vi "GeoData.vi"() -> ()   [LabVIEW 2017] (continued)
Washington Parish\tH1\n71075\t22119\tSpringhill\tLA\tWebster Parish\tH1\n71067\t22119\tPrinceton\tLA\tWebster Parish\tH1\n71071\t22119\tSarepta\tLA\tWebster Parish\tH1\n71038\t22119\tHaynesville\tLA\tWebster Parish\tH1\n71073\t22119\tSibley\tLA\tWebster Parish\tH1\n71024\t22119\tDubberly\tLA\tWebster Parish\tH1\n71055\t22119\tMinden\tLA\tWebster Parish\tH1\n71072\t22119\tShongaloo\tLA\tWebster Parish\tH1\n71039\t22119\tHeflin\tLA\tWebster Parish\tH1\n71037\t22119\tHaughton\tLA\tWebster Parish\tH1\n71023\t22119\tDoyline\tLA\tWebster Parish\tH1\n71021\t22119\tCullen\tLA\tWebster Parish\tH1\n71018\t22119\tCotton valley\tLA\tWebster Parish\tH1\n70773\t22121\tRougon\tLA\tWest Baton Rouge Parish\tH1\n70710\t22121\tAddis\tLA\tWest Baton Rouge Parish\tH1\n70764\t22121\tPlaquemine\tLA\tWest Baton Rouge Parish\tH1\n70736\t22121\tGlynn\tLA\tWest Baton Rouge Parish\tH1\n70719\t22121\tBrusly\tLA\tWest Baton Rouge Parish\tH1\n70767\t22121\tPort allen\tLA\tWest Baton Rouge Parish\tH1\n70729\t22121\tErwinville\tLA\tWest Baton Rouge Parish\tH1\n71263\t22123\tOak grove\tLA\tWest Carroll Parish\tH1\n71269\t22123\tRayville\tLA\tWest Carroll Parish\tH1\n71286\t22123\tTransylvania\tLA\tWest Carroll Parish\tH1\n71253\t22123\tKilbourne\tLA\tWest Carroll Parish\tH1\n71266\t22123\tPioneer\tLA\tWest Carroll Parish\tH1\n71237\t22123\tEpps\tLA\tWest Carroll Parish\tH1\n71242\t22123\tForest\tLA\tWest Carroll Parish\tH1\n70748\t22125\tJackson\tLA\tWest Feliciana Parish\tH1\n70787\t22125\tWeyanoke\tLA\tWest Feliciana Parish\tH1\n70775\t22125\tSaint francisville\tLA\tWest Feliciana Parish\tH1\n70712\t22125\tAngola\tLA\tWest Feliciana Parish\tH1\n70784\t22125\tWakefield\tLA\tWest Feliciana Parish\tH1\n70782\t22125\tTunica\tLA\tWest Feliciana Parish\tH1\n71070\t22127\tSaline\tLA\tWinn Parish\tH1\n71483\t22127\tWinnfield\tLA\tWinn Parish\tH1\n71479\t22127\tTullos\tLA\tWinn Parish\tH1\n71465\t22127\tOlla\tLA\tWinn Parish\tH1\n71471\t22127\tSaint maurice\tLA\tWinn Parish\tH1\n71457\t22127\tNatchitoches\tLA\tWinn Parish\tH1\n71031\t22127\tGoldonna\tLA\tWinn Parish\tH1\n71422\t22127\tDodson\tLA\tWinn Parish\tH1\n71404\t22127\tAtlanta\tLA\tWinn Parish\tH1\n71454\t22127\tMontgomery\tLA\tWinn Parish\tH1\n71432\t22127\tGeorgetown\tLA\tWinn Parish\tH1\n71473\t22127\tSikes\tLA\tWinn Parish\tH1\n71440\t22127\tJoyce\tLA\tWinn Parish\tH1\n71410\t22127\tCalvin\tLA\tWinn Parish\tH1\n4212\t23001\tAuburn\tME\tAndroscoggin County\tH1\n4220\t23001\tBuckfield\tME\tAndroscoggin County\tH1\n4240\t23001\tLewiston\tME\tAndroscoggin County\tH1\n4274\t23001\tPoland\tME\tAndroscoggin County\tH1\n4270\t23001\tOxford\tME\tAndroscoggin County\tH1\n4256\t23001\tMechanic falls\tME\tAndroscoggin County\tH1\n4239\t23001\tJay\tME\tAndroscoggin County\tH1\n4230\t23001\tEast poland\tME\tAndroscoggin County\tH1\n4228\t23001\tEast livermore\tME\tAndroscoggin County\tH1\n4210\t23001\tAuburn\tME\tAndroscoggin County\tH1\n4222\t23001\tDurham\tME\tAndroscoggin County\tH1\n4254\t23001\tLivermore falls\tME\tAndroscoggin County\tH1\n4252\t23001\tLisbon falls\tME\tAndroscoggin County\tH1\n4211\t23001\tAuburn\tME\tAndroscoggin County\tH1\n4238\t23001\tHebron\tME\tAndroscoggin County\tH1\n4266\t23001\tNorth turner\tME\tAndroscoggin County\tH1\n4288\t23001\tWest minot\tME\tAndroscoggin County\tH1\n4260\t23001\tNew gloucester\tME\tAndroscoggin County\tH1\n4250\t23001\tLisbon\tME\tAndroscoggin County\tH1\n4280\t23001\tSabattus\tME\tAndroscoggin County\tH1\n4263\t23001\tLeeds\tME\tAndroscoggin County\tH1\n4253\t23001\tLivermore\tME\tAndroscoggin County\tH1\n4243\t23001\tLewiston\tME\tAndroscoggin County\tH1\n4282\t23001\tTurner\tME\tAndroscoggin County\tH1\n4258\t23001\tMinot\tME\tAndroscoggin County\tH1\n4291\t23001\tWest poland\tME\tAndroscoggin County\tH1\n4223\t23001\tDanville\tME\tAndroscoggin County\tH1\n4236\t23001\tGreene\tME\tAndroscoggin County\tH1\n4241\t23001\tLewiston\tME\tAndroscoggin County\tH1\n4487\t23003\tSpringfield\tME\tAroostook County\tH1\n4739\t23003\tEagle lake\tME\tAroostook County\tH1\n4733\t23003\tBenedicta\tME\tAroostook County\tH1\n4775\t23003\tSheridan\tME\tAroostook County\tH1\n4762\t23003\tNew sweden\tME\tAroostook County\tH1\n4459\t23003\tMattawamkeag\tME\tAroostook County\tH1\n4777\t23003\tStacyville\tME\tAroostook County\tH1\n4761\t23003\tNew limerick\tME\tAroostook County\tH1\n4750\t23003\tLimestone\tME\tAroostook County\tH1\n4787\t23003\tWestfield\tME\tAroostook County\tH1\n4740\t23003\tEaston\tME\tAroostook County\tH1\n4746\t23003\tGrand isle\tME\tAroostook County\tH1\n4763\t23003\tOakfield\tME\tAroostook County\tH1\n4776\t23003\tSherman\tME\tAroostook County\tH1\n4738\t23003\tCrouseville\tME\tAroostook County\tH1\n4772\t23003\tSaint agatha\tME\tAroostook County\tH1\n4764\t23003\tOxbow\tME\tAroostook County\tH1\n4745\t23003\tFrenchville\tME\tAroostook County\tH1\n4424\t23003\tDanforth\tME\tAroostook County\tH1\n4742\t23003\tFort fairfield\tME\tAroostook County\tH1\n4736\t23003\tCaribou\tME\tAroostook County\tH1\n4756\t23003\tMadawaska\tME\tAroostook County\tH1\n4779\t23003\tSinclair\tME\tAroostook County\tH1\n4783\t23003\tStockholm\tME\tAroostook County\tH1\n4751\t23003\tLimestone\tME\tAroostook County\tH1\n4735\t23003\tBridgewater\tME\tAroostook County\tH1\n4732\t23003\tAshland\tME\tAroostook County\tH1\n4743\t23003\tFort kent\tME\tAroostook County\tH1\n4757\t23003\tMapleton\tME\tAroostook County\tH1\n4786\t23003\tWashburn\tME\tAroostook County\tH1\n4769\t23003\tPresque isle\tME\tAroostook County\tH1\n4781\t23003\tWallagrass\tME\tAroostook County\tH1\n4451\t23003\tKingman\tME\tAroostook County\tH1\n4747\t23003\tIsland falls\tME\tAroostook County\tH1\n4768\t23003\tPortage\tME\tAroostook County\tH1\n4744\t23003\tFort kent mills\tME\tAroostook County\tH1\n4737\t23003\tClayton lake\tME\tAroostook County\tH1\n4497\t23003\tWytopitlock\tME\tAroostook County\tH1\n4730\t23003\tHoulton\tME\tAroostook County\tH1\n4758\t23003\tMars hill\tME\tAroostook County\tH1\n4471\t23003\tOrient\tME\tAroostook County\tH1\n4766\t23003\tPerham\tME\tAroostook County\tH1\n4773\t23003\tSaint david\tME\tAroostook County\tH1\n4760\t23003\tMonticello\tME\tAroostook County\tH1\n4785\t23003\tVan buren\tME\tAroostook County\tH1\n4780\t23003\tSmyrna mills\tME\tAroostook County\tH1\n4774\t23003\tSaint francis\tME\tAroostook County\tH1\n4734\t23003\tBlaine\tME\tAroostook County\tH1\n4062\t23005\tWindham\tME\tCumberland County\tH1\n4015\t23005\tCasco\tME\tCumberland County\tH1\n4093\t23005\tBuxton\tME\tCumberland County\tH1\n4109\t23005\tPortland\tME\tCumberland County\tH1\n4274\t23005\tPoland\tME\tCumberland County\tH1\n4078\t23005\tSouth freeport\tME\tCumberland County\tH1\n4082\t23005\tSouth windham\tME\tCumberland County\tH1\n4071\t23005\tRaymond\tME\tCumberland County\tH1\n4088\t23005\tWaterford\tME\tCumberland County\tH1\n4069\t23005\tPownal\tME\tCumberland County\tH1\n4098\t23005\tWestbrook\tME\tCumberland County\tH1\n4091\t23005\tWest baldwin\tME\tCumberland County\tH1\n4021\t23005\tCumberland center\tME\tCumberland County\tH1\n4222\t23005\tDurham\tME\tCumberland County\tH1\n4066\t23005\tOrrs island\tME\tCumberland County\tH1\n4034\t23005\tFreeport\tME\tCumberland County\tH1\n4033\t23005\tFreeport\tME\tCumberland County\tH1\n4040\t23005\tHarrison\tME\tCumberland County\tH1\n4096\t23005\tYarmouth\tME\tCumberland County\tH1\n4074\t23005\tScarborough\tME\tCumberland County\tH1\n4103\t23005\tPortland\tME\tCumberland County\tH1\n4105\t23005\tFalmouth\tME\tCumberland County\tH1\n4108\t23005\tPeaks island\tME\tCumberland County\tH1\n4110\t23005\tCumberland foreside\tME\tCumberland County\tH1\n4085\t23005\tSteep falls\tME\tCumberland County\tH1\n4123\t23005\tPortland\tME\tCumberland County\tH1\n4009\t23005\tBridgton\tME\tCumberland County\tH1\n4092\t23005\tWestbrook\tME\tCumberland County\tH1\n4079\t23005\tHarpswell\tME\tCumberland County\tH1\n4102\t23005\tPortland\tME\tCumberland County\tH1\n4097\t23005\tNorth yarmouth\tME\tCumberland County\tH1\n4038\t23005\tGorham\tME\tCumberland County\tH1\n4039\t23005\tGray\tME\tCumberland County\tH1\n4029\t23005\tSebago\tME\tCumberland County\tH1\n4101\t23005\tPortland\tME\tCumberland County\tH1\n4260\t23005\tNew gloucester\tME\tCumberland County\tH1\n4017\t23005\tChebeague island\tME\tCumberland County\tH1\n4070\t23005\tScarborough\tME\tCumberland County\tH1\n4116\t23005\tSouth portland\tME\tCumberland County\tH1\n4057\t23005\tNorth bridgton\tME\tCumberland County\tH1\n4077\t23005\tSouth casco\tME\tCumberland County\tH1\n4055\t23005\tNaples\tME\tCumberland County\tH1\n4106\t23005\tSouth portland\tME\tCumberland County\tH1\n4107\t23005\tCape elizabeth\tME\tCumberland County\tH1\n4122\t23005\tPortland\tME\tCumberland County\tH1\n4024\t23005\tEast baldwin\tME\tCumberland County\tH1\n4124\t23005\tPortland\tME\tCumberland County\tH1\n4013\t23005\tBustins island\tME\tCumberland County\tH1\n4019\t23005\tCliff island\tME\tCumberland County\tH1\n4050\t23005\tLong island\tME\tCumberland County\tH1\n4011\t23005\tBrunswick\tME\tCumberland County\tH1\n4032\t23005\tFreeport\tME\tCumberland County\tH1\n4064\t23005\tOld orchard beach\tME\tCumberland County\tH1\n4084\t23005\tStandish\tME\tCumberland County\tH1\n4112\t23005\tPortland\tME\tCumberland County\tH1\n4003\t23005\tBailey island\tME\tCumberland County\tH1\n4104\t23005\tPortland\tME\tCumberland County\tH1\n4984\t23007\tTemple\tME\tFranklin County\tH1\n4262\t23007\tNorth jay\tME\tFranklin County\tH1\n4225\t23007\tDryden\tME\tFranklin County\tH1\n4940\t23007\tFarmington falls\tME\tFranklin County\tH1\n4294\t23007\tWilton\tME\tFranklin County\tH1\n4239\t23007\tJay\tME\tFranklin County\tH1\n4966\t23007\tPhillips\tME\tFranklin County\tH1\n4938\t23007\tFarmington\tME\tFranklin County\tH1\n4285\t23007\tWeld\tME\tFranklin County\tH1\n4970\t23007\tRangeley\tME\tFranklin County\tH1\n4964\t23007\tOquossoc\tME\tFranklin County\tH1\n4961\t23007\tNew portland\tME\tFranklin County\tH1\n4983\t23007\tStrong\tME\tFranklin County\tH1\n4956\t23007\tNew vineyard\tME\tFranklin County\tH1\n4234\t23007\tEast wilton\tME\tFranklin County\tH1\n4224\t23007\tDixfield\tME\tFranklin County\tH1\n4227\t23007\tEast dixfield\tME\tFranklin County\tH1\n4982\t23007\tStratton\tME\tFranklin County\tH1\n4992\t23007\tWest farmington\tME\tFranklin County\tH1\n4955\t23007\tNew sharon\tME\tFranklin County\tH1\n4947\t23007\tKingfield\tME\tFranklin County\tH1\n4936\t23007\tEustis\tME\tFranklin County\tH1\n4616\t23009\tBrooklin\tME\tHancock County\tH1\n4660\t23009\tMount desert\tME\tHancock County\tH1\n4642\t23009\tHarborside\tME\tHancock County\tH1\n4646\t23009\tIslesford\tME\tHancock County\tH1\n4609\t23009\tBar harbor\tME\tHancock County\tH1\n4622\t23009\tCherryfield\tME\tHancock County\tH1\n4677\t23009\tSorrento\tME\tHancock County\tH1\n4408\t23009\tAurora\tME\tHancock County\tH1\n4679\t23009\tSouthwest harbor\tME\tHancock County\tH1\n4612\t23009\tBernard\tME\tHancock County\tH1\n4669\t23009\tProspect harbor\tME\tHancock County\tH1\n4629\t23009\tEast blue hill\tME\tHancock County\tH1\n4676\t23009\tSedgwick\tME\tHancock County\tH1\n4674\t23009\tSeal cove\tME\tHancock County\tH1\n4614\t23009\tBlue hill\tME\tHancock County\tH1\n4617\t23009\tBrooksville\tME\tHancock County\tH1\n4607\t23009\tGouldsboro\tME\tHancock County\tH1\n4673\t23009\tSargentville\tME\tHancock County\tH1\n4624\t23009\tCorea\tME\tHancock County\tH1\n4416\t23009\tBucksport\tME\tHancock County\tH1\n4476\t23009\tPenobscot\tME\tHancock County\tH1\n4684\t23009\tSurry\tME\tHancock County\tH1\n4675\t23009\tSeal harbor\tME\tHancock County\tH1\n4613\t23009\tBirch harbor\tME\tHancock County\tH1\n4650\t23009\tLittle deer isle\tME\tHancock County\tH1\n4431\t23009\tEast orland\tME\tHancock County\tH1\n4627\t23009\tDeer isle\tME\tHancock County\tH1\n4640\t23009\tHancock\tME\tHancock County\tH1\n4653\t23009\tBass harbor\tME\tHancock County\tH1\n4685\t23009\tSwans island\tME\tHancock County\tH1\n4644\t23009\tHulls cove\tME\tHancock County\tH1\n4672\t23009\tSalsbury cove\tME\tHancock County\tH1\n4605\t23009\tEllsworth\tME\tHancock County\tH1\n4681\t23009\tStonington\tME\tHancock County\tH1\n4421\t23009\tCastine\tME\tHancock County\tH1\n4664\t23009\tSullivan\tME\tHancock County\tH1\n4625\t23009\tCranberry isles\tME\tHancock County\tH1\n4429\t23009\tHolden\tME\tHancock County\tH1\n4472\t23009\tOrland\tME\tHancock County\tH1\n4634\t23009\tFranklin\tME\tHancock County\tH1\n4420\t23009\tCastine\tME\tHancock County\tH1\n4683\t23009\tSunset\tME\tHancock County\tH1\n4693\t23009\tWinter harbor\tME\tHancock County\tH1\n4662\t23009\tNortheast harbor\tME\tHancock County\tH1\n4635\t23009\tFrenchboro\tME\tHancock County\tH1\n4345\t23011\tGardiner\tME\tKennebec County\tH1\n4338\t23011\tAugusta\tME\tKennebec County\tH1\n4918\t23011\tBelgrade lakes\tME\tKennebec County\tH1\n4935\t23011\tEast vassalboro\tME\tKennebec County\tH1\n4353\t23011\tWhitefield\tME\tKennebec County\tH1\n4333\t23011\tAugusta\tME\tKennebec County\tH1\n4254\t23011\tLivermore falls\tME\tKennebec County\tH1\n4287\t23011\tBowdoin\tME\tKennebec County\tH1\n4364\t23011\tWinthrop\tME\tKennebec County\tH1\n4350\t23011\tLitchfield\tME\tKennebec County\tH1\n4346\t23011\tRandolph\tME\tKennebec County\tH1\n4910\t23011\tAlbion\tME\tKennebec County\tH1\n4989\t23011\tVassalboro\tME\tKennebec County\tH1\n4937\t23011\tFairfield\tME\tKennebec County\tH1\n4359\t23011\tSouth gardiner\tME\tKennebec County\tH1\n4284\t23011\tWayne\tME\tKennebec County\tH1\n4926\t23011\tChina village\tME\tKennebec County\tH1\n4351\t23011\tManchester\tME\tKennebec County\tH1\n4988\t23011\tUnity\tME\tKennebec County\tH1\n4927\t23011\tClinton\tME\tKennebec County\tH1\n4259\t23011\tMonmouth\tME\tKennebec County\tH1\n4363\t23011\tWindsor\tME\tKennebec County\tH1\n4355\t23011\tReadfield\tME\tKennebec County\tH1\n4360\t23011\tVienna\tME\tKennebec County\tH1\n4901\t23011\tWaterville\tME\tKennebec County\tH1\n4332\t23011\tAugusta\tME\tKennebec County\tH1\n4349\t23011\tKents hill\tME\tKennebec County\tH1\n4903\t23011\tWaterville\tME\tKennebec County\tH1\n4962\t23011\tNorth vassalboro\tME\tKennebec County\tH1\n4357\t23011\tRichmond\tME\tKennebec County\tH1\n4358\t23011\tSouth china\tME\tKennebec County\tH1\n4963\t23011\tOakland\tME\tKennebec County\tH1\n4978\t23011\tSmithfield\tME\tKennebec County\tH1\n4352\t23011\tMount vernon\tME\tKennebec County\tH1\n4265\t23011\tNorth monmouth\tME\tKennebec County\tH1\n4343\t23011\tEast winthrop\tME\tKennebec County\tH1\n4336\t23011\tAugusta\tME\tKennebec County\tH1\n4330\t23011\tAugusta\tME\tKennebec County\tH1\n4344\t23011\tFarmingdale\tME\tKennebec County\tH1\n4347\t23011\tHallowell\tME\tKennebec County\tH1\n4917\t23011\tBelgrade\tME\tKennebec County\tH1\n4856\t23013\tRockport\tME\tKnox County\tH1\n4949\t23013\tLiberty\tME\tKnox County\tH1\n4547\t23013\tFriendship\tME\tKnox County\tH1\n4847\t23013\tHope\tME\tKnox County\tH1\n4863\t23013\tVinalhaven\tME\tKnox County\tH1\n4865\t23013\tWest rockport\tME\tKnox County\tH1\n4860\t23013\tTenants harbor\tME\tKnox County\tH1\n4843\t23013\tCamden\tME\tKnox County\tH1\n4853\t23013\tNorth haven\tME\tKnox County\tH1\n4572\t23013\tWaldoboro\tME\tKnox County\tH1\n4563\t23013\tCushing\tME\tKnox County\tH1\n4862\t23013\tUnion\tME\tKnox County\tH1\n4574\t23013\tWashington\tME\tKnox County\tH1\n4645\t23013\tIsle au haut\tME\tKnox County\tH1\n4841\t23013\tRockland\tME\tKnox County\tH1\n4861\t23013\tThomaston\tME\tKnox County\tH1\n4855\t23013\tPort clyde\tME\tKnox County\tH1\n4858\t23013\tSouth thomaston\tME\tKnox County\tH1\n4851\t23013\tMatinicus\tME\tKnox County\tH1\n4854\t23013\tOwls head\tME\tKnox County\tH1\n4864\t23013\tWarren\tME\tKnox County\tH1\n4859\t23013\tSpruce head\tME\tKnox County\tH1\n4539\t23015\tBristol\tME\tLincoln County\tH1\n4543\t23015\tDamariscotta\tME\tLincoln County\tH1\n4348\t23015\tJefferson\tME\tLincoln County\tH1\n4353\t23015\tWhitefield\tME\tLincoln County\tH1\n4556\t23015\tEdgecomb\tME\tLincoln County\tH1\n4342\t23015\tDresden\tME\tLincoln County\tH1\n4554\t23015\tNew harbor\tME\tLincoln County\tH1\n4571\t23015\tTrevett\tME\tLincoln County\tH1\n4575\t23015\tWest boothbay harbor\tME\tLincoln County\tH1\n4852\t23015\tMonhegan\tME\tLincoln County\tH1\n4535\t23015\tAlna\tME\tLincoln County\tH1\n4570\t23015\tSquirrel island\tME\tLincoln County\tH1\n4537\t23015\tBoothbay\tME\tLincoln County\tH1\n4541\t23015\tChamberlain\tME\tLincoln County\tH1\n4544\t23015\tEast boothbay\tME\tLincoln County\tH1\n4573\t23015\tWalpole\tME\tLincoln County\tH1\n4354\t23015\tPalermo\tME\tLincoln County\tH1\n4572\t23015\tWaldoboro\tME\tLincoln County\tH1\n4862\t23015\tUnion\tME\tLincoln County\tH1\n4551\t23015\tBremen\tME\tLincoln County\tH1\n4558\t23015\tPemaquid\tME\tLincoln County\tH1\n4538\t23015\tBoothbay harbor\tME\tLincoln County\tH1\n4555\t23015\tNobleboro\tME\tLincoln County\tH1\n4568\t23015\tSouth bristol\tME\tLincoln County\tH1\n4576\t23015\tSouthport\tME\tLincoln County\tH1\n4564\t23015\tRound pond\tME\tLincoln County\tH1\n4341\t23015\tCoopers mills\tME\tLincoln County\tH1\n4553\t23015\tNewcastle\tME\tLincoln County\tH1\n4578\t23015\tWiscasset\tME\tLincoln County\tH1\n4864\t23015\tWarren\tME\tLincoln County\tH1\n4220\t23017\tBuckfield\tME\tOxford County\tH1\n4276\t23017\tRumford\tME\tOxford County\tH1\n4268\t23017\tNorway\tME\tOxford County\tH1\n4270\t23017\tOxford\tME\tOxford County\tH1\n4275\t23017\tRoxbury\tME\tOxford County\tH1\n4226\t23017\tEast andover\tME\tOxford County\tH1\n4267\t23017\tNorth waterford\tME\tOxford County\tH1\n4016\t23017\tCenter lovell\tME\tOxford County\tH1\n4051\t23017\tLovell\tME\tOxford County\tH1\n4088\t23017\tWaterford\tME\tOxford County\tH1\n4239\t23017\tJay\tME\tOxford County\tH1\n4221\t23017\tCanton\tME\tOxford County\tH1\n4261\t23017\tNewry\tME\tOxford County\tH1\n4041\t23017\tHiram\tME\tOxford County\tH1\n4289\t23017\tWest paris\tME\tOxford County\tH1\n4040\t23017\tHarrison\tME\tOxford County\tH1\n4224\t23017\tDixfield\tME\tOxford County\tH1\n4231\t23017\tStoneham\tME\tOxford County\tH1\n4292\t23017\tSumner\tME\tOxford County\tH1\n4238\t23017\tHebron\tME\tOxford County\tH1\n4009\t23017\tBridgton\tME\tOxford County\tH1\n4257\t23017\tMexico\tME\tOxford County\tH1\n4290\t23017\tPeru\tME\tOxford County\tH1\n4219\t23017\tBryant pond\tME\tOxford County\tH1\n4216\t23017\tAndover\tME\tOxford County\tH1\n4217\t23017\tBethel\tME\tOxford County\tH1\n4255\t23017\tGreenwood\tME\tOxford County\tH1\n4237\t23017\tHanover\tME\tOxford County\tH1\n4271\t23017\tParis\tME\tOxford County\tH1\n4037\t23017\tFryeburg\tME\tOxford County\tH1\n4258\t23017\tMinot\tME\tOxford County\tH1\n4010\t23017\tBrownfield\tME\tOxford County\tH1\n4022\t23017\tDenmark\tME\tOxford County\tH1\n4068\t23017\tPorter\tME\tOxford County\tH1\n4281\t23017\tSouth paris\tME\tOxford County\tH1\n4286\t23017\tWest bethel\tME\tOxford County\tH1\n4487\t23019\tSpringfield\tME\tPenobscot County\tH1\n4444\t23019\tHampden\tME\tPenobscot County\tH1\n4434\t23019\tEtna\tME\tPenobscot County\tH1\n4417\t23019\tBurlington\tME\tPenobscot County\tH1\n4469\t23019\tOrono\tME\tPenobscot County\tH1\n4765\t23019\tPatten\tME\tPenobscot County\tH1\n4733\t23019\tBenedicta\tME\tPenobscot County\tH1\n4493\t23019\tWest enfield\tME\tPenobscot County\tH1\n4460\t23019\tMedway\tME\tPenobscot County\tH1\n4932\t23019\tDixmont\tME\tPenobscot County\tH1\n4928\t23019\tCorinna\tME\tPenobscot County\tH1\n4455\t23019\tLee\tME\tPenobscot County\tH1\n4459\t23019\tMattawamkeag\tME\tPenobscot County\tH1\n4777\t23019\tStacyville\tME\tPenobscot County\tH1\n4410\t23019\tBradford\tME\tPenobscot County\tH1\n4474\t23019\tOrrington\tME\tPenobscot County\tH1\n4930\t23019\tDexter\tME\tPenobscot County\tH1\n4450\t23019\tKenduskeag\tME\tPenobscot County\tH1\n4495\t23019\tWinn\tME\tPenobscot County\tH1\n4412\t23019\tBrewer\tME\tPenobscot County\tH1\n4435\t23019\tExeter\tME\tPenobscot County\tH1\n4473\t23019\tOrono\tME\tPenobscot County\tH1\n4457\t23019\tLincoln\tME\tPenobscot County\tH1\n4953\t23019\tNewport\tME\tPenobscot County\tH1\n4419\t23019\tCarmel\tME\tPenobscot County\tH1\n4488\t23019\tStetson\tME\tPenobscot County\tH1\n4411\t23019\tBradley\tME\tPenobscot County\tH1\n4401\t23019\tBangor\tME\tPenobscot County\tH1\n4453\t23019\tLagrange\tME\tPenobscot County\tH1\n4462\t23019\tMillinocket\tME\tPenobscot County\tH1\n4489\t23019\tStillwater\tME\tPenobscot County\tH1\n4933\t23019\tEast newport\tME\tPenobscot County\tH1\n4422\t23019\tCharleston\tME\tPenobscot County\tH1\n4402\t23019\tBangor\tME\tPenobscot County\tH1\n4468\t23019\tOld town\tME\tPenobscot County\tH1\n4461\t23019\tMilford\tME\tPenobscot County\tH1\n4939\t23019\tGarland\tME\tPenobscot County\tH1\n4430\t23019\tEast millinocket\tME\tPenobscot County\tH1\n4451\t23019\tKingman\tME\tPenobscot County\tH1\n4449\t23019\tHudson\tME\tPenobscot County\tH1\n4497\t23019\tWytopitlock\tME\tPenobscot County\tH1\n4428\t23019\tEddington\tME\tPenobscot County\tH1\n4456\t23019\tLevant\tME\tPenobscot County\tH1\n4969\t23019\tPlymouth\tME\tPenobscot County\tH1\n4475\t23019\tPassadumkeag\tME\tPenobscot County\tH1\n4418\t23019\tGreenbush\tME\tPenobscot County\tH1\n4429\t23019\tHolden\tME\tPenobscot County\tH1\n4921\t23019\tBrooks\tME\tPenobscot County\tH1\n4427\t23019\tCorinth\tME\tPenobscot County\tH1\n4448\t23019\tHowland\tME\tPenobscot County\tH1\n4426\t23021\tDover foxcroft\tME\tPiscataquis County\tH1\n4415\t23021\tBrownville junction\tME\tPiscataquis County\tH1\n4942\t23021\tHarmony\tME\tPiscataquis County\tH1\n4930\t23021\tDexter\tME\tPiscataquis County\tH1\n4481\t23021\tSebec\tME\tPiscataquis County\tH1\n4414\t23021\tBrownville\tME\tPiscataquis County\tH1\n4479\t23021\tSangerville\tME\tPiscataquis County\tH1\n4464\t23021\tMonson\tME\tPiscataquis County\tH1\n4485\t23021\tShirley mills\tME\tPiscataquis County\tH1\n4463\t23021\tMilo\tME\tPiscataquis County\tH1\n4441\t23021\tGreenville\tME\tPiscataquis County\tH1\n4442\t23021\tGreenville junction\tME\tPiscataquis County\tH1\n4443\t23021\tGuilford\tME\tPiscataquis County\tH1\n4406\t23021\tAbbot\tME\tPiscataquis County\tH1\n4448\t23021\tHowland\tME\tPiscataquis County\tH1\n4345\t23023\tGardiner\tME\tSagadahoc County\tH1\n4086\t23023\tTopsham\tME\tSagadahoc County\tH1\n4562\t23023\tPhippsburg\tME\tSagadahoc County\tH1\n4008\t23023\tBowdoinham\tME\tSagadahoc County\tH1\n4565\t23023\tSebasco estates\tME\tSagadahoc County\tH1\n4252\t23023\tLisbon falls\tME\tSagadahoc County\tH1\n4287\t23023\tBowdoin\tME\tSagadahoc County\tH1\n4548\t23023\tGeorgetown\tME\tSagadahoc County\tH1\n4530\t23023\tBath\tME\tSagadahoc County\tH1\n4357\t23023\tRichmond\tME\tSagadahoc County\tH1\n4011\t23023\tBrunswick\tME\tSagadahoc County\tH1\n4579\t23023\tWoolwich\tME\tSagadahoc County\tH1\n4942\t23025\tHarmony\tME\tSomerset County\tH1\n4967\t23025\tPittsfield\tME\tSomerset County\tH1\n4938\t23025\tFarmington\tME\tSomerset County\tH1\n4924\t23025\tCanaan\tME\tSomerset County\tH1\n4976\t23025\tSkowhegan\tME\tSomerset County\tH1\n4930\t23025\tDexter\tME\tSomerset County\tH1\n4961\t23025\tNew portland\tME\tSomerset County\tH1\n4937\t23025\tFairfield\tME\tSomerset County\tH1\n4923\t23025\tCambridge\tME\tSomerset County\tH1\n4911\t23025\tAnson\tME\tSomerset County\tH1\n4957\t23025\tNorridgewock\tME\tSomerset County\tH1\n4945\t23025\tJackman\tME\tSomerset County\tH1\n4912\t23025\tAthens\tME\tSomerset County\tH1\n4950\t23025\tMadison\tME\tSomerset County\tH1\n4927\t23025\tClinton\tME\tSomerset County\tH1\n4925\t23025\tCaratunk\tME\tSomerset County\tH1\n4954\t23025\tNew portland\tME\tSomerset County\tH1\n4920\t23025\tBingham\tME\tSomerset County\tH1\n4943\t23025\tHartland\tME\tSomerset County\tH1\n4955\t23025\tNew sharon\tME\tSomerset County\tH1\n4985\t23025\tWest forks\tME\tSomerset County\tH1\n4478\t23025\tRockwood\tME\tSomerset County\tH1\n4978\t23025\tSmithfield\tME\tSomerset County\tH1\n4965\t23025\tPalmyra\tME\tSomerset County\tH1\n4971\t23025\tSaint albans\tME\tSomerset County\tH1\n4975\t23025\tShawmut\tME\tSomerset County\tH1\n4929\t23025\tDetroit\tME\tSomerset County\tH1\n4958\t23025\tNorth anson\tME\tSomerset County\tH1\n4979\t23025\tSolon\tME\tSomerset County\tH1\n4944\t23025\tHinckley\tME\tSomerset County\tH1\n4438\t23027\tFrankfort\tME\tWaldo County\tH1\n4915\t23027\tBelfast\tME\tWaldo County\tH1\n4949\t23027\tLiberty\tME\tWaldo County\tH1\n4848\t23027\tIslesboro\tME\tWaldo County\tH1\n4952\t23027\tMorrill\tME\tWaldo County\tH1\n4973\t23027\tSearsmont\tME\tWaldo County\tH1\n4981\t23027\tStockton springs\tME\tWaldo County\tH1\n4974\t23027\tSearsport\tME\tWaldo County\tH1\n4986\t23027\tThorndike\tME\tWaldo County\tH1\n4496\t23027\tWinterport\tME\tWaldo County\tH1\n4951\t23027\tMonroe\tME\tWaldo County\tH1\n4354\t23027\tPalermo\tME\tWaldo County\tH1\n4922\t23027\tBurnham\tME\tWaldo County\tH1\n4988\t23027\tUnity\tME\tWaldo County\tH1\n4941\t23027\tFreedom\tME\tWaldo County\tH1\n4987\t23027\tTroy\tME\tWaldo County\tH1\n4850\t23027\tLincolnville center\tME\tWaldo County\tH1\n4358\t23027\tSouth china\tME\tWaldo County\tH1\n4849\t23027\tLincolnville\tME\tWaldo County\tH1\n4921\t23027\tBrooks\tME\tWaldo County\tH1\n4619\t23029\tCalais\tME\tWashington County\tH1\n4628\t23029\tDennysville\tME\tWashington County\tH1\n4643\t23029\tHarrington\tME\tWashington County\tH1\n4658\t23029\tMilbridge\tME\tWashington County\tH1\n4666\t23029\tPembroke\tME\tWashington County\tH1\n4652\t23029\tLubec\tME\tWashington County\tH1\n4622\t23029\tCherryfield\tME\tWashington County\tH1\n4606\t23029\tAddison\tME\tWashington County\tH1\n4657\t23029\tMeddybemps\tME\tWashington County\tH1\n4649\t23029\tJonesport\tME\tWashington County\tH1\n4668\t23029\tPrinceton\tME\tWashington County\tH1\n4413\t23029\tBrookton\tME\tWashington County\tH1\n4492\t23029\tWaite\tME\tWashington County\tH1\n4626\t23029\tCutler\tME\tWashington County\tH1\n4490\t23029\tTopsfield\tME\tWashington County\tH1\n4611\t23029\tBeals\tME\tWashington County\tH1\n4424\t23029\tDanforth\tME\tWashington County\tH1\n4631\t23029\tEastport\tME\tWashington County\tH1\n4667\t23029\tPerry\tME\tWashington County\tH1\n4694\t23029\tBaileyville\tME\tWashington County\tH1\n4671\t23029\tRobbinston\tME\tWashington County\tH1\n4491\t23029\tVanceboro\tME\tWashington County\tH1\n4654\t23029\tMachias\tME\tWashington County\tH1\n4623\t23029\tColumbia falls\tME\tWashington County\tH1\n4691\t23029\tWhiting\tME\tWashington County\tH1\n4454\t23029\tLambert lake\tME\tWashington County\tH1\n4630\t23029\tEast machias\tME\tWashington County\tH1\n4648\t23029\tJonesboro\tME\tWashington County\tH1\n4680\t23029\tSteuben\tME\tWashington County\tH1\n4655\t23029\tMachiasport\tME\tWashington County\tH1\n4686\t23029\tWesley\tME\tWashington County\tH1\n4637\t23029\tGrand lake stream\tME\tWashington County\tH1\n3901\t23031\tBerwick\tME\tYork County\tH1\n4001\t23031\tActon\tME\tYork County\tH1\n3904\t23031\tKittery\tME\tYork County\tH1\n4043\t23031\tKennebunk\tME\tYork County\tH1\n4030\t23031\tEast waterboro\tME\tYork County\tH1\n4093\t23031\tBuxton\tME\tYork County\tH1\n4054\t23031\tMoody\tME\tYork County\tH1\n3902\t23031\tCape neddick\tME\tYork County\tH1\n4027\t23031\tLebanon\tME\tYork County\tH1\n4047\t23031\tParsonsfield\tME\tYork County\tH1\n4042\t23031\tHollis center\tME\tYork County\tH1\n3906\t23031\tNorth berwick\tME\tYork County\tH1\n3908\t23031\tSouth berwick\tME\tYork County\tH1\n4061\t23031\tNorth waterboro\tME\tYork County\tH1\n4083\t23031\tSpringvale\tME\tYork County\tH1\n4095\t23031\tWest newfield\tME\tYork County\tH1\n4028\t23031\tEast parsonsfield\tME\tYork County\tH1\n4006\t23031\tBiddeford pool\tME\tYork County\tH1\n3804\t23031\tPortsmouth\tME\tYork County\tH1\n4002\t23031\tAlfred\tME\tYork County\tH1\n3910\t23031\tYork beach\tME\tYork County\tH1\n4049\t23031\tLimington\tME\tYork County\tH1\n4074\t23031\tScarborough\tME\tYork County\tH1\n4076\t23031\tShapleigh\tME\tYork County\tH1\n4087\t23031\tWaterboro\tME\tYork County\tH1\n4056\t23031\tNewfield\tME\tYork County\tH1\n4014\t23031\tCape porpoise\tME\tYork County\tH1\n4020\t23031\tCornish\tME\tYork County\tH1\n3905\t23031\tKittery point\tME\tYork County\tH1\n3907\t23031\tOgunquit\tME\tYork County\tH1\n3909\t23031\tYork\tME\tYork County\tH1\n4038\t23031\tGorham\tME\tYork County\tH1\n4048\t23031\tLimerick\tME\tYork County\tH1\n4073\t23031\tSanford\tME\tYork County\tH1\n4063\t23031\tOcean park\tME\tYork County\tH1\n4094\t23031\tWest kennebunk\tME\tYork County\tH1\n4005\t23031\tBiddeford\tME\tYork County\tH1\n4046\t23031\tKennebunkport\tME\tYork County\tH1\n4072\t23031\tSaco\tME\tYork County\tH1\n4090\t23031\tWells\tME\tYork County\tH1\n4004\t23031\tBar mills\tME\tYork County\tH1\n3903\t23031\tEliot\tME\tYork County\tH1\n3911\t23031\tYork harbor\tME\tYork County\tH1\n4064\t23031\tOld orchard beach\tME\tYork County\tH1\n4084\t23031\tStandish\tME\tYork County\tH1\n21529\t24001\tEllerslie\tMD\tAllegany County\tH1\n21562\t24001\tWesternport\tMD\tAllegany County\tH1\n21540\t24001\tLuke\tMD\tAllegany County\tH1\n21766\t24001\tLittle orleans\tMD\tAllegany County\tH1\n21521\t24001\tBarton\tMD\tAllegany County\tH1\n21542\t24001\tMidland\tMD\tAllegany County\tH1\n21503\t24001\tCumberland\tMD\tAllegany County\tH1\n21556\t24001\tPinto\tMD\tAllegany County\tH1\n21504\t24001\tCumberland\tMD\tAllegany County\tH1\n21528\t24001\tEckhart mines\tMD\tAllegany County\tH1\n21532\t24001\tFrostburg\tMD\tAllegany County\tH1\n21560\t24001\tSpring gap\tMD\tAllegany County\tH1\n21530\t24001\tFlintstone\tMD\tAllegany County\tH1\n21555\t24001\tOldtown\tMD\tAllegany County\tH1\n21750\t24001\tHancock\tMD\tAllegany County\tH1\n21524\t24001\tCorriganville\tMD\tAllegany County\tH1\n21505\t24001\tCumberland\tMD\tAllegany County\tH1\n21502\t24001\tCumberland\tMD\tAllegany County\tH1\n21539\t24001\tLonaconing\tMD\tAllegany County\tH1\n21501\t24001\tCumberland\tMD\tAllegany County\tH1\n21557\t24001\tRawlings\tMD\tAllegany County\tH1\n21543\t24001\tMidlothian\tMD\tAllegany County\tH1\n21545\t24001\tMount savage\tMD\tAllegany County\tH1\n20779\t24003\tTracys landing\tMD\tAnne Arundel County\tH1\n21144\t24003\tSevern\tMD\tAnne Arundel County\tH1\n21240\t24003\tBaltimore\tMD\tAnne Arundel County\tH1\n21405\t24003\tAnnapolis\tMD\tAnne Arundel County\tH1\n20714\t24003\tNorth beach\tMD\tAnne Arundel County\tH1\n20736\t24003\tOwings\tMD\tAnne Arundel County\tH1\n21412\t24003\tAnnapolis\tMD\tAnne Arundel County\tH1\n21106\t24003\tMayo\tMD\tAnne Arundel County\tH1\n20733\t24003\tChurchton\tMD\tAnne Arundel County\tH1\n21037\t24003\tEdgewater\tMD\tAnne Arundel County\tH1\n21060\t24003\tGlen burnie\tMD\tAnne Arundel County\tH1\n21108\t24003\tMillersville\tMD\tAnne Arundel County\tH1\n21114\t24003\tCrofton\tMD\tAnne Arundel County\tH1\n21404\t24003\tAnnapolis\tMD\tAnne Arundel County\tH1\n21411\t24003\tAnnapolis\tMD\tAnne Arundel County\tH1\n20724\t24003\tLaurel\tMD\tAnne Arundel County\tH1\n20751\t24003\tDeale\tMD\tAnne Arundel County\tH1\n20794\t24003\tJessup\tMD\tAnne Arundel County\tH1\n21054\t24003\tGambrills\tMD\tAnne Arundel County\tH1\n21122\t24003\tPasadena\tMD\tAnne Arundel County\tH1\n21403\t24003\tAnnapolis\tMD\tAnne Arundel County\tH1\n20711\t24003\tLothian\tMD\tAnne Arundel County\tH1\n21032\t24003\tCrownsville\tMD\tAnne Arundel County\tH1\n21226\t24003\tCurtis bay\tMD\tAnne Arundel County\tH1\n21056\t24003\tGibson island\tMD\tAnne Arundel County\tH1\n20776\t24003\tHarwood\tMD\tAnne Arundel County\tH1\n21012\t24003\tArnold\tMD\tAnne Arundel County\tH1\n21140\t24003\tRiva\tMD\tAnne Arundel County\tH1\n21401\t24003\tAnnapolis\tMD\tAnne Arundel County\tH1\n21409\t24003\tAnnapolis\tMD\tAnne Arundel County\tH1\n20758\t24003\tFriendship\tMD\tAnne Arundel County\tH1\n21402\t24003\tAnnapolis\tMD\tAnne Arundel County\tH1\n21077\t24003\tHarmans\tMD\tAnne Arundel County\tH1\n20754\t24003\tDunkirk\tMD\tAnne Arundel County\tH1\n20764\t24003\tShady side\tMD\tAnne Arundel County\tH1\n20778\t24003\tWest river\tMD\tAnne Arundel County\tH1\n21061\t24003\tGlen burnie\tMD\tAnne Arundel County\tH1\n21076\t24003\tHanover\tMD\tAnne Arundel County\tH1\n20701\t24003\tAnnapolis junction\tMD\tAnne Arundel County\tH1\n20755\t24003\tFort george g meade\tMD\tAnne Arundel County\tH1\n21035\t24003\tDavidsonville\tMD\tAnne Arundel County\tH1\n21090\t24003\tLinthicum heights\tMD\tAnne Arundel County\tH1\n21113\t24003\tOdenton\tMD\tAnne Arundel County\tH1\n21146\t24003\tSeverna park\tMD\tAnne Arundel County\tH1\n21225\t24003\tBrooklyn\tMD\tAnne Arundel County\tH1\n21123\t24003\tPasadena\tMD\tAnne Arundel County\tH1\n20765\t24003\tGalesville\tMD\tAnne Arundel County\tH1\n21062\t24003\tGlen burnie\tMD\tAnne Arundel County\tH1\n21043\t24005\tEllicott city\tMD\tBaltimore County\tH1\n21022\t24005\tBrooklandville\tMD\tBaltimore County\tH1\n21093\t24005\tLutherville timonium\tMD\tBaltimore County\tH1\n21162\t24005\tWhite marsh\tMD\tBaltimore County\tH1\n21207\t24005\tGwynn oak\tMD\tBaltimore County\tH1\n21210\t24005\tBaltimore\tMD\tBaltimore County\tH1\n21237\t24005\tRosedale\tMD\tBaltimore County\tH1\n21282\t24005\tPikesville\tMD\tBaltimore County\tH1\n21027\t24005\tChase\tMD\tBaltimore County\tH1\n21020\t24005\tBoring\tMD\tBaltimore County\tH1\n21031\t24005\tHunt valley\tMD\tBaltimore County\tH1\n21053\t24005\tFreeland\tMD\tBaltimore County\tH1\n21057\t24005\tGlen arm\tMD\tBaltimore County\tH1\n21087\t24005\tKingsville\tMD\tBaltimore County\tH1\n21074\t24005\tHampstead\tMD\tBaltimore County\tH1\n21128\t24005\tPerry hall\tMD\tBaltimore County\tH1\n21152\t24005\tSparks glencoe\tMD\tBaltimore County\tH1\n21221\t24005\tEssex\tMD\tBaltimore County\tH1\n21234\t24005\tParkville\tMD\tBaltimore County\tH1\n21236\t24005\tNottingham\tMD\tBaltimore County\tH1\n21156\t24005\tUpper falls\tMD\tBaltimore County\tH1\n21284\t24005\tTowson\tMD\tBaltimore County\tH1\n21092\t24005\tLong green\tMD\tBaltimore County\tH1\n21136\t24005\tReisterstown\tMD\tBaltimore County\tH1\n21071\t24005\tGlyndon\tMD\tBaltimore County\tH1\n21102\t24005\tManchester\tMD\tBaltimore County\tH1\n21133\t24005\tRandallstown\tMD\tBaltimore County\tH1\n21206\t24005\tBaltimore\tMD\tBaltimore County\tH1\n21222\t24005\tDundalk\tMD\tBaltimore County\tH1\n21228\t24005\tCatonsville\tMD\tBaltimore County\tH1\n21229\t24005\tBaltimore\tMD\tBaltimore County\tH1\n21250\t24005\tBaltimore\tMD\tBaltimore County\tH1\n21065\t24005\tHunt valley\tMD\tBaltimore County\tH1\n21030\t24005\tCockeysville\tMD\tBaltimore County\tH1\n21085\t24005\tJoppa\tMD\tBaltimore County\tH1\n21111\t24005\tMonkton\tMD\tBaltimore County\tH1\n21209\t24005\tBaltimore\tMD\tBaltimore County\tH1\n21212\t24005\tBaltimore\tMD\tBaltimore County\tH1\n21219\t24005\tSparrows point\tMD\tBaltimore County\tH1\n21153\t24005\tStevenson\tMD\tBaltimore County\tH1\n21023\t24005\tButler\tMD\tBaltimore County\tH1\n21105\t24005\tMaryland line\tMD\tBaltimore County\tH1\n21094\t24005\tLutherville timonium\tMD\tBaltimore County\tH1\n21117\t24005\tOwings mills\tMD\tBaltimore County\tH1\n21163\t24005\tWoodstock\tMD\tBaltimore County\tH1\n21208\t24005\tPikesville\tMD\tBaltimore County\tH1\n21220\t24005\tMiddle river\tMD\tBaltimore County\tH1\n21131\t24005\tPhoenix\tMD\tBaltimore County\tH1\n21082\t24005\tHydes\tMD\tBaltimore County\tH1\n21241\t24005\tBaltimore\tMD\tBaltimore County\tH1\n21051\t24005\tFork\tMD\tBaltimore County\tH1\n21120\t24005\tParkton\tMD\tBaltimore County\tH1\n21161\t24005\tWhite hall\tMD\tBaltimore County\tH1\n21215\t24005\tBaltimore\tMD\tBaltimore County\tH1\n21224\t24005\tBaltimore\tMD\tBaltimore County\tH1\n21227\t24005\tHalethorpe\tMD\tBaltimore County\tH1\n21239\t24005\tBaltimore\tMD\tBaltimore County\tH1\n21286\t24005\tTowson\tMD\tBaltimore County\tH1\n21155\t24005\tUpperco\tMD\tBaltimore County\tH1\n21235\t24005\tBaltimore\tMD\tBaltimore County\tH1\n21252\t24005\tTowson\tMD\tBaltimore County\tH1\n21013\t24005\tBaldwin\tMD\tBaltimore County\tH1\n21204\t24005\tTowson\tMD\tBaltimore County\tH1\n21225\t24005\tBrooklyn\tMD\tBaltimore County\tH1\n21244\t24005\tWindsor mill\tMD\tBaltimore County\tH1\n21104\t24005\tMarriottsville\tMD\tBaltimore County\tH1\n21052\t24005\tFort howard\tMD\tBaltimore County\tH1\n21139\t24005\tRiderwood\tMD\tBaltimore County\tH1\n21285\t24005\tTowson\tMD\tBaltimore County\tH1\n20678\t24009\tPrince frederick\tMD\tCalvert County\tH1\n20714\t24009\tNorth beach\tMD\tCalvert County\tH1\n20736\t24009\tOwings\tMD\tCalvert County\tH1\n20688\t24009\tSolomons\tMD\tCalvert County\tH1\n20610\t24009\tBarstow\tMD\tCalvert County\tH1\n20639\t24009\tHuntingtown\tMD\tCalvert County\tH1\n20615\t24009\tBroomes island\tMD\tCalvert County\tH1\n20657\t24009\tLusby\tMD\tCalvert County\tH1\n20732\t24009\tChesapeake beach\tMD\tCalvert County\tH1\n20676\t24009\tPort republic\tMD\tCalvert County\tH1\n20758\t24009\tFriendship\tMD\tCalvert County\tH1\n20685\t24009\tSaint leonard\tMD\tCalvert County\tH1\n20754\t24009\tDunkirk\tMD\tCalvert County\tH1\n20629\t24009\tDowell\tMD\tCalvert County\tH1\n20689\t24009\tSunderland\tMD\tCalvert County\tH1\n21636\t24011\tGoldsboro\tMD\tCaroline County\tH1\n21639\t24011\tGreensboro\tMD\tCaroline County\tH1\n21640\t24011\tHenderson\tMD\tCaroline County\tH1\n21649\t24011\tMarydel\tMD\tCaroline County\tH1\n21655\t24011\tPreston\tMD\tCaroline County\tH1\n21657\t24011\tQueen anne\tMD\tCaroline County\tH1\n21629\t24011\tDenton\tMD\tCaroline County\tH1\n21660\t24011\tRidgely\tMD\tCaroline County\tH1\n21641\t24011\tHillsboro\tMD\tCaroline County\tH1\n21609\t24011\tBethlehem\tMD\tCaroline County\tH1\n21632\t24011\tFederalsburg\tMD\tCaroline County\tH1\n21643\t24011\tHurlock\tMD\tCaroline County\tH1\n21757\t24013\tKeymar\tMD\tCarroll County\tH1\n21074\t24013\tHampstead\tMD\tCarroll County\tH1\n21771\t24013\tMount airy\tMD\tCarroll County\tH1\n21784\t24013\tSykesville\tMD\tCarroll County\tH1\n21787\t24013\tTaneytown\tMD\tCarroll County\tH1\n21157\t24013\tWestminster\tMD\tCarroll County\tH1\n21158\t24013\tWestminster\tMD\tCarroll County\tH1\n21136\t24013\tReisterstown\tMD\tCarroll County\tH1\n21102\t24013\tManchester\tMD\tCarroll County\tH1\n21048\t24013\tFinksburg\tMD\tCarroll County\tH1\n21776\t24013\tNew windsor\tMD\tCarroll County\tH1\n21791\t24013\tUnion bridge\tMD\tCarroll County\tH1\n21155\t24013\tUpperco\tMD\tCarroll County\tH1\n21797\t24013\tWoodbine\tMD\tCarroll County\tH1\n21104\t24013\tMarriottsville\tMD\tCarroll County\tH1\n21914\t24015\tCharlestown\tMD\tCecil County\tH1\n21920\t24015\tElk mills\tMD\tCecil County\tH1\n21922\t24015\tElkton\tMD\tCecil County\tH1\n21903\t24015\tPerryville\tMD\tCecil County\tH1\n21921\t24015\tElkton\tMD\tCecil County\tH1\n21911\t24015\tRising sun\tMD\tCecil County\tH1\n21913\t24015\tCecilton\tMD\tCecil County\tH1\n21904\t24015\tPort deposit\tMD\tCecil County\tH1\n21901\t24015\tNorth east\tMD\tCecil County\tH1\n21915\t24015\tChesapeake city\tMD\tCecil County\tH1\n21917\t24015\tColora\tMD\tCecil County\tH1\n21930\t24015\tGeorgetown\tMD\tCecil County\tH1\n21912\t24015\tWarwick\tMD\tCecil County\tH1\n21916\t24015\tChilds\tMD\tCecil County\tH1\n21919\t24015\tEarleville\tMD\tCecil County\tH1\n21902\t24015\tPerry point\tMD\tCecil County\tH1\n21918\t24015\tConowingo\tMD\tCecil County\tH1\n20693\t24017\tWelcome\tMD\tCharles County\tH1\n20662\t24017\tNanjemoy\tMD\tCharles County\tH1\n20617\t24017\tBryantown\tMD\tCharles County\tH1\n20625\t24017\tCobb island\tMD\tCharles County\tH1\n20659\t24017\tMechanicsville\tMD\tCharles County\tH1\n20640\t24017\tIndian head\tMD\tCharles County\tH1\n20645\t24017\tIssue\tMD\tCharles County\tH1\n20622\t24017\tCharlotte hall\tMD\tCharles County\tH1\n20646\t24017\tLa plata\tMD\tCharles County\tH1\n20643\t24017\tIronsides\tMD\tCharles County\tH1\n20664\t24017\tNewburg\tMD\tCharles County\tH1\n20658\t24017\tMarbury\tMD\tCharles County\tH1\n20611\t24017\tBel alton\tMD\tCharles County\tH1\n20695\t24017\tWhite plains\tMD\tCharles County\tH1\n20675\t24017\tPomfret\tMD\tCharles County\tH1\n20661\t24017\tMount victoria\tMD\tCharles County\tH1\n20603\t24017\tWaldorf\tMD\tCharles County\tH1\n20602\t24017\tWaldorf\tMD\tCharles County\tH1\n20677\t24017\tPort tobacco\tMD\tCharles County\tH1\n20604\t24017\tWaldorf\tMD\tCharles County\tH1\n20601\t24017\tWaldorf\tMD\tCharles County\tH1\n20637\t24017\tHughesville\tMD\tCharles County\tH1\n20612\t24017\tBenedict\tMD\tCharles County\tH1\n20632\t24017\tFaulkner\tMD\tCharles County\tH1\n20607\t24017\tAccokeek\tMD\tCharles County\tH1\n20613\t24017\t
